vi "WorkorderHandler_getDataToModify(StoreLocked).vi"(0 "reference":T1, 3 "timeout in ms (-1)":i32=-1, 5 "error in (no error)":errorcluster) -> (14 "duplicate reference":T1, 16 "data":T2, 18 "timed out?":bool, 19 "error out":errorcluster)   [LabVIEW 2011]
doc: "Returns the data of dqGOOP object and locks it. In addition, this function stores the locked data in a cache so it is available for the getData(Locked) function."
uses:
  DataStructures/WorkorderHandler_ObjectReference.ctl
  DataStructures/WorkorderHandler_ObjectData.ctl
panel:
  in  "queue (default)":refnum<queue>
  # "Copyright (C) 2004 DataAct Incorporated"
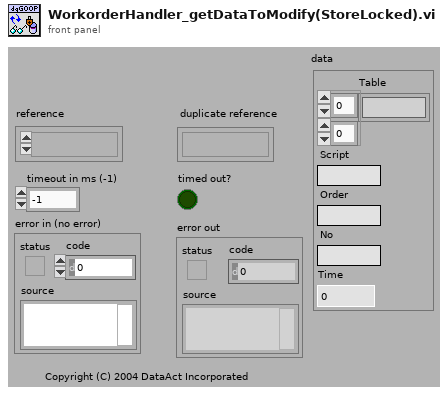
[diagram p1: front panel]
types:
  T1 = typedef "WorkorderHandler_ObjectReference.ctl" = refnum<k1>
  T2 = typedef "WorkorderHandler_ObjectData.ctl" = cluster{"Table":string[][], "Script":string, "Order":string, "No":string, "Time":dbl}
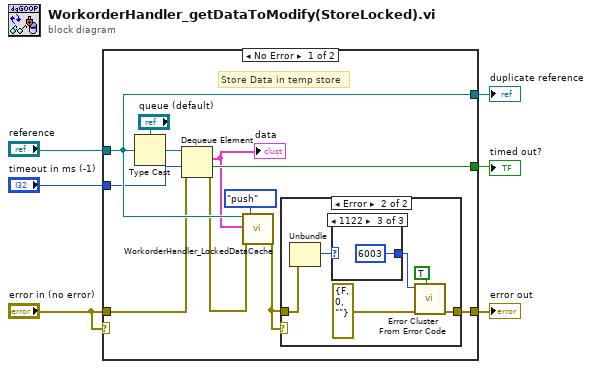
[diagram p0: block diagram]
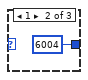
[diagram p4: hidden frame]
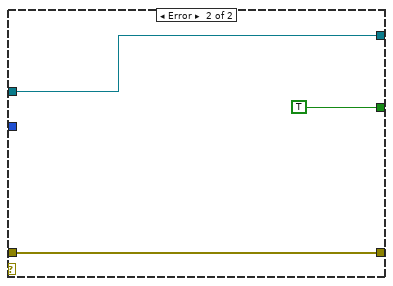
[diagram p5: hidden frame]
diagram:
  n1 = case shown="No Error" "error in (no error)" {
    tunnel: [w15 w28] -> w6
    tunnel: [w17 TRUE] -> w1
    tunnel: "reference" -> [w14 w29]
    tunnel: [w14 w29] -> w4
    tunnel: "timeout in ms (-1)" -> [w7 _]
    tunnel: "error in (no error)" -> [w11 w28]
    frame No Error {
      # "Store Data in temp store"
      n2 = Type Cast(type="queue (default)", x=w14) -> (*(type *) &x=w12:refnum<queue>)
      n3 = Dequeue Element(queue=w12, timeout in ms (-1)=w7, error in (no error)=w11) -> (element=w8:T2, timed out?=w17:bool, error out=w10:errorcluster)  [unwired: 1 out]
      "data" <- w8
      n4 = call "WorkorderHandler_LockedDataCache.vi"("reference"=w14, "data in"=w8, "error in (no error)"=w10, "action (read)"=enum16{"push", "read", "pop"}."push" ("action")) -> ("error out"=w9:errorcluster)  [unwired: 15 out]
      n5 = case shown="Error" w9 {
        tunnel: [w18 w19] -> w15
        tunnel: w9 -> [w18 w24]
        frame No Error {
        }
        frame Error {
          n6 = Unbundle(w24) -> ("code"=w23:i32)  [unwired: 2 out]
          n7 = case shown="1122" w23 {
            selector: w23 -> [w25 _ _]
            tunnel: [w25 6004 ("code") 6003 ("code")] -> w21
            frame Default {
            }
            frame 1 {
            }
            frame 1122 {
            }
          }
          n8 = call <vilib>:"Error Cluster From Error Code.vi"("show call chain? (False)"=TRUE, "error in (no error)"=errorcluster {"status"=FALSE, "code"=0, "source"=""} ("error out"), "error code (0)"=w21) -> ("error out"=w19:errorcluster)  [unwired: 6 out]
        }
      }
    }
    frame Error {
    }
  }
  "error out" <- w6
  "duplicate reference" <- w4
  "timed out?" <- w1
